vi "Write SysCfg Device Object.vi"(8 "error in":errorcluster, 10 "Device Information":T1 {"Product ID" format="%.0x"}, 11 "SysCfg Device in":refnum<class "SysCfg Device.lvclass">) -> (0 "error out":errorcluster, 3 "SysCfg Device out":refnum<class "SysCfg Device.lvclass">)   [LabVIEW 2015, in "SMI.lvlib" / "SysCfg Device.lvclass"]
uses:
  SysCfg Device.lvclass
  Controls/SysCfgDeviceInformation.ctl
  SysCfg Device.lvclass/SysCfg Device.ctl
  Device/Device.lvclass/Device.ctl
  Write SysCfg Session.vi
  Device/Accessor Methods/Write Vendor Name.vi
  Device/Accessor Methods/Write Product Name.vi
  Device/Accessor Methods/Write Product ID.vi
  Device/Accessor Methods/Write Serial Number.vi
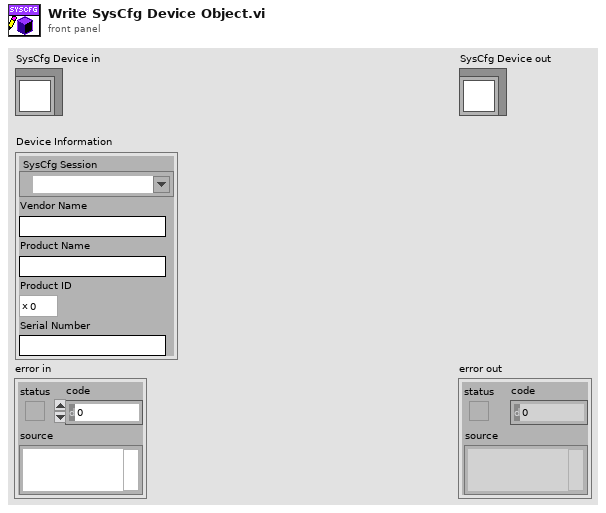
[diagram p1: front panel]
types:
  T1 = typedef "SMI.lvlib/SysCfg Device.lvclass/SysCfgDeviceInformation.ctl" = cluster{"SysCfg Session":refnum<k21>, "Vendor Name":string, "Product Name":string, "Product ID":u32, "Serial Number":string}
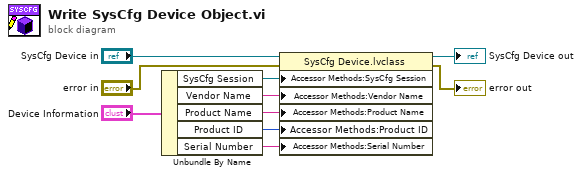
[diagram p0: block diagram]
diagram:
  n1 = Unbundle By Name("Device Information") -> ("SysCfg Session"=w7:refnum<k21>, "Vendor Name"=w6:string, "Product Name"=w5:string, "Product ID"=w4:u32, "Serial Number"=w3:string)
  n2 = property class="SysCfg Device.lvclass"(reference="SysCfg Device in", error in="error in", "Accessor Methods:SysCfg Session"=w7, "Accessor Methods:Vendor Name"=w6, "Accessor Methods:Product Name"=w5, "Accessor Methods:Product ID"=w4, "Accessor Methods:Serial Number"=w3) -> (reference out=→"SysCfg Device out":refnum<class "SysCfg Device.lvclass">, error out=→"error out":errorcluster)
